vi "Hexa to Double.vi"(0 "Hexa":string, 1 "Index":i32) -> (5 "Double":dbl)   [LabVIEW 2017]
doc: "Long aus Trackerantwort (Hexa)\n\nIndex: \n0 = Size\n4 = Datatype\n8 = Command \n12 = Result Status"
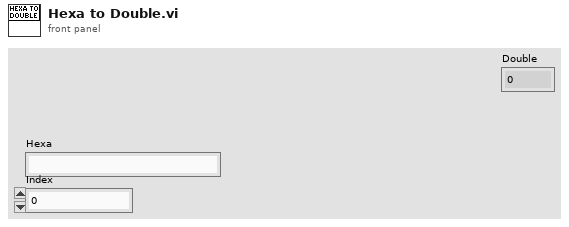
[diagram p1: front panel]
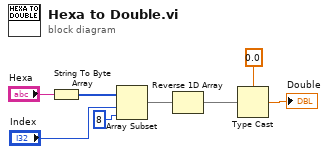
[diagram p0: block diagram]
diagram:
  n1 = String To Byte Array(string="Hexa") -> (unsigned byte array=w8:u8[])
  n2 = Array Subset(array=w8, index="Index", length=8 ("Länge")) -> (w7:u8[])
  n3 = Reverse 1D Array(array=w7) -> (reversed array=w6:u8[])
  n4 = Type Cast(type=0.0, x=w6) -> (*(type *) &x=→"Double":dbl)
